vi "InterfaceTest.vi"() -> ()   [LabVIEW 2017]
uses:
  Interface/Configuration.ctl
  <vilib>/rvi/Analysis/control/PID/Typedef/niFpgaPID_PIGains.ctl
  <vilib>/rvi/Analysis/control/PID/Typedef/niFpgaPID_OutputRange.ctl
  FPGA/HarmonicFilter.ctl
  <instrlib>/_niInstr/FIFO Register Bus/v1/Host/niInstr FIFO Register Bus v1 Host.lvclass
  C:/Program Files (x86)/National Instruments/LabVIEW 2017/instr.lib/_niInstr/Instruction Framework/v1/Host/Instruction Target/niInstr Instruction Target v1 Host.lvclass
  <vilib>/FPGAPlugInAG/sbRIO-9607/niLvFpga_Open_sbRIO-9607.vi
  <vilib>/rvi/interface/common/dynamic/niFpgaDynamicAddResources.vi
  <vilib>/FPGAPlugInAG/Dynamic/niLvFpga_Reset_Dynamic.vi
  <vilib>/FPGAPlugInAG/Dynamic/niLvFpga_Run_Dynamic.vi
  <vilib>/Utility/error.llb/Error Cluster From Error Code.vi
  <vilib>/rvi/errors/niLvFpgaAdjustHostInterfaceError.vi
  <vilib>/rvi/interface/nirviOpenFPGA/nirviOpenFPGA.xnode
  FPGA Bitfiles/ThreePhasePLLdev_FPGATarget_IFwTest_AXdVPM-7ZFk.lvbitx
  FPGA/IFwTest.vi
  <vilib>/rvi/interface/nirviMethod/nirviMethod.xnode
  <vilib>/rvi/interface/nirviReadWriteControl/nirviReadWriteControl.xnode
  Interface/ThreePhasePLLInterface.lvlib
  NiFpgaLv.dll
  <vilib>/rvi/interface/Simulation/niFpgaSimulationCallBeginRW.vi
  FPGA/ThreePhasePLL.lvlib
panel:
  out "detectedFreq":sgl
  out "IsLocked":bool
  out "HarmonicFilter":cluster{"ak":sgl, "bk":sgl}
  in  "Configuration":T1={"PLLgains"={"proportional gain"=1.0, "integral gain"=2.0}, "PLLrange"={"output high (Inf)"=3.0, "output low (-Inf)"=4.0}, "dT"=5.0, "expectedFreq"=20.0, "lockDuration"=7.0, "freqBoundaries"=8.0, "HarmonicFilter"={"enable"=TRUE, "coeff"={"ak"=9.0, "bk"=10.0}}} {"PLLgains"."proportional gain" step=0.125}
  out "dT":sgl
  out "lockDuration":u32
  out "expectedFreq":sgl
  out "freqBoundary":sgl
  out "reset":bool
  out "PLLRange":T5
  out "PLLGains":T6
  in  "locked":bool
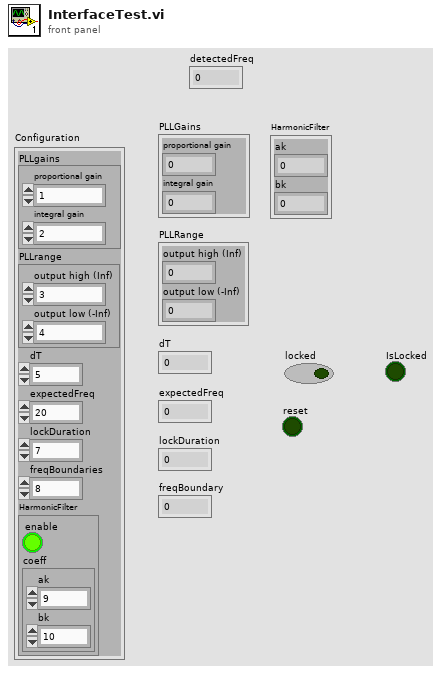
[diagram p1: front panel]
types:
  T1 = typedef "ThreePhasePLLInterface.lvlib/Configuration.ctl" = cluster{"PLLgains":T2, "PLLrange":T3, "dT":sgl, "expectedFreq":sgl, "lockDuration":sgl, "freqBoundaries":sgl, "HarmonicFilter":cluster{"enable":bool, "coeff":T4}}
  T2 = typedef "niFpgaPID_PIGains.ctl" = cluster{"proportional gain":sgl, "integral gain":sgl}
  T3 = typedef "niFpgaPID_OutputRange.ctl" = cluster{"output high (Inf)":sgl, "output low (-Inf)":sgl}
  T4 = typedef "ThreePhasePLL.lvlib/HarmonicFilter.ctl" = cluster{"ak":sgl, "bk":sgl}
  T5 = cluster{"output high (Inf)":sgl, "output low (-Inf)":sgl}
  T6 = cluster{"proportional gain":sgl, "integral gain":sgl}
  T7 = typedef "ThreePhasePLLInterface.lvlib/InterfaceRef.ctl" = cluster{"instruction target":refnum<class "niInstr Instruction Target v1 Host.lvclass">, "context":refnum<class "niInstr Instruction Framework Context v1 Host.lvclass">}
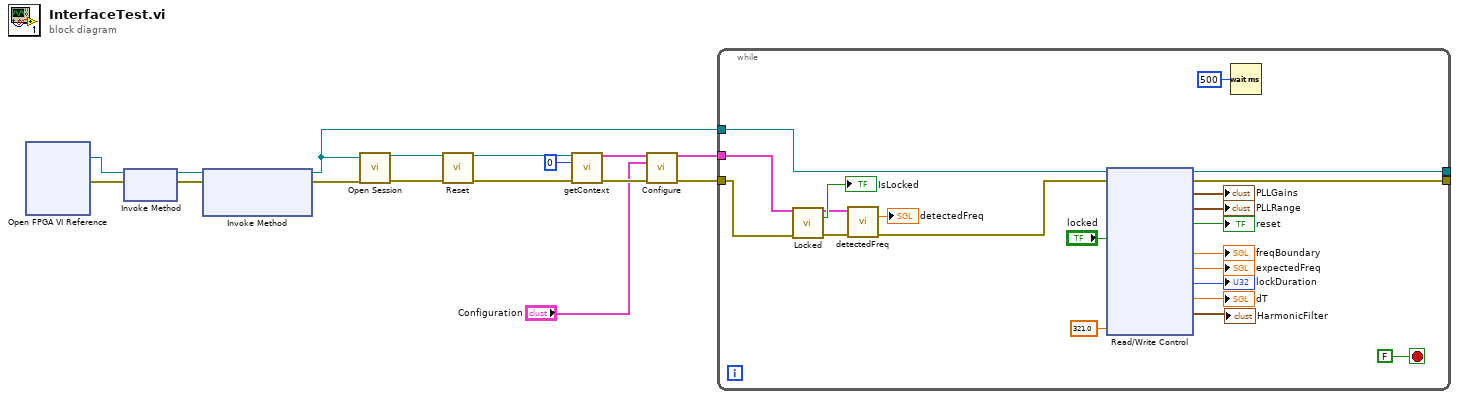
[diagram p0: block diagram]
diagram:
  n1 = xnode "Open FPGA VI Reference"() -> ("FPGA VI Reference Out"=w10:refnum<k20>, "error out"=w11:errorcluster)  [unwired: 2 in]
  n2 = xnode "Invoke Method"("FPGA VI Reference In"=w10, "error in"=w11) -> ("FPGA VI Reference Out"=w14:refnum<k20>, "error out"=w13:errorcluster)
  n3 = xnode "Invoke Method"("FPGA VI Reference In"=w14, "error in"=w13) -> ("FPGA VI Reference Out"=w4:refnum<k20>, "error out"=w12:errorcluster)  [unwired: 1 in]
  n4 = call <instrlib>:"Open Session.vi"("fpga ref"=w4, "error in"=w12) -> ("session out"=w15:refnum<class "niInstr FIFO Register Bus v1 Host.lvclass">, "error out"=w16:errorcluster)  [unwired: 12 in]
  n5 = call-dynamic "Reset.vi"("session in"=w15, "error in"=w16) -> ("session out"=w9:refnum<class "niInstr FIFO Register Bus v1 Host.lvclass">, "error out"=w8:errorcluster)  [unwired: 12 in]
  n6 = call "getContext.vi"("instruction target in"=w9, "instance"=u8 0, "error in"=w8) -> ("Interface"=w6:T7, "error out"=w5:errorcluster)  [unwired: 11 in]
  n7 = call "Configure.vi"("Interface in"=w6, "Configuration"="Configuration", "error in"=w5) -> ("Interface out"=w2:T7, "error out"=w3:errorcluster)  [unwired: 11 in]
  n8 = while {
    tunnel: w4 -> [w37]
    tunnel: w3 -> [w23]
    tunnel: w2 -> [w24]
    tunnel: [w35] -> _
    tunnel: [w34] -> _
    stop <- FALSE stop-if-true
    n9 = call "Locked.vi"("Interface in"=w24, "error in"=w23) -> ("Interface out"=w20:T7, "Locked"=→"IsLocked":bool, "error out"=w19:errorcluster)  [unwired: 11 in]
    n10 = call "detectedFreq.vi"("Interface in"=w20, "error in"=w19) -> ("detectedFreq"=→"detectedFreq":sgl, "error out"=w17:errorcluster)  [unwired: 11 in, 1 out]
    n11 = xnode "Read/Write Control"("FPGA VI Reference In"=w37, "error in"=w17, "locked"="locked", "detectedFreq"=sgl 321.0) -> ("FPGA VI Reference Out"=w35:refnum<k20>, "error out"=w34:errorcluster, "PLLGains"=→"PLLGains":T6, "PLLRange"=→"PLLRange":T5, "reset"=→"reset":bool, "freqBoundary"=→"freqBoundary":sgl, "expectedFreq"=→"expectedFreq":sgl, "lockDuration"=→"lockDuration":u32, "dT"=→"dT":sgl, "HarmonicFilter"=→"HarmonicFilter":cluster{"ak":sgl, "bk":sgl})
    n12 = Wait (ms)(milliseconds to wait=u32 500) -> ()  [unwired: 1 out]
  }
